vi "ATM.vi"() -> ()   [LabVIEW 2021]
doc: "This is the Main VI that performs the AMT operations."
uses:
  Controls/Queue_Operation_Select.ctl
  Controls/State_Data.ctl
  Controls/Control_Reference.ctl
  Controls/File_Operation_Select.ctl
  Controls/Timer_Operation_Select.ctl
  Controls/ATM_Data.ctl
  Controls/Right_Menu_Display.ctl
  Controls/Left_Menu_Dispaly.ctl
  Controls/Notifier_Operation_Select.ctl
  Controls/ATM_Message.ctl
panel:
  in  "User_Input":string caption="User Input"
  out "Error_Out":errorcluster
  in  "Error_In":errorcluster
  out "ATM_Message":string caption="ATM Message"
  out "Right_Menu":T1 caption="Right Menu"
  out "Left_Menu":T2 caption="Left Menu"
  in  "Right_Buttons":T3 caption="Right Buttons"
  in  "Left_Buttons":T4 caption="Left Buttons"
  in  "Enter":bool
  in  "Card_Simulator":bool caption="Card Simulator"
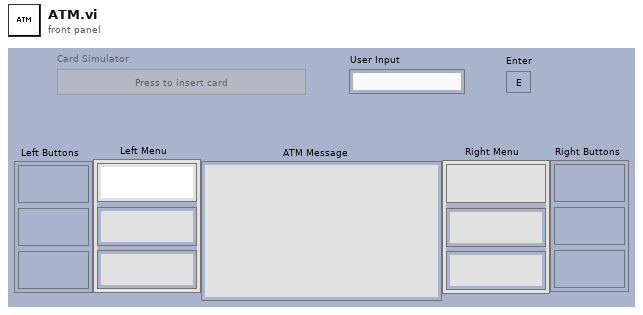
[diagram p1: front panel]
types:
  T1 = typedef "Right_Menu_Display.ctl" = cluster{"Withdraw_D":string, "Deposit_D":string, "Fast_cash_$50_D":string}
  T2 = typedef "Left_Menu_Dispaly.ctl" = cluster{"Balance_Inquiry_D":string, "None_D":string, "Return_Card_&_Terminate":string}
  T3 = cluster{"Deposit":bool, "Withdraw":bool, "Fast_Cash_$50":bool}
  T4 = cluster{"None":bool, "Balance_Inquiry":bool, "Return_Card_&_Terminate":bool}
  T5 = typedef "Notifier_Operation_Select.ctl" = enum16{"Obtain_Notification", "Send_Notification", "Get_Notification_Status", "Release_Notification"}
  T6 = typedef "Queue_Operation_Select.ctl" = enum16{"Obtain_Queue", "Enqueue", "Enqueue_N", "Enqueue_at_First", "Dequeue", "Flush_Queue", "Release_Queue"}
  T7 = typedef "Timer_Operation_Select.ctl" = enum16{"Start_Timer", "Time_Out?", "Stop_Timer"}
  T8 = typedef "State_Data.ctl" = cluster{"State":string, "Data":string}
  T9 = typedef "ATM_Data.ctl" = cluster{"Account_Details":string[][], "Selected_Account_Details":string[], "ATM_Message":string, "Left_Menu":T2, "Right_Menu":T1, "Contol_Buttons":refnum<vi>[], "Enter_&_User_Input":refnum<vi>[], "Card_Simulator":refnum<vi>[], "Disable_Control_Reference":refnum<vi>[], "Enable_Control_Reference":refnum<vi>[], "Control_Reference":T10, "Current_Process":string, "Event_Data":string, "Current_Banking_Process":string, "Selected_Banking":string, "Index_of_Selected_Account":i32, "Terminated?":bool, "Account_File_Path":path, "ATM_Message 2":T11}
  T10 = typedef "Control_Reference.ctl" = cluster{"User_Input":refnum<vi>, "Fast_Cash_$50":refnum<vi>, "Withdraw":refnum<vi>, "Deposit":refnum<vi>, "Return_Card_&_Terminate":refnum<vi>, "Balance_Inquiry":refnum<vi>, "None":refnum<vi>, "Enter":refnum<vi>, "Card_Simulator":refnum<vi>}
  T11 = typedef "ATM_Message.ctl" = cluster{"LM_Balance_Inquiry":string, "LM_None":string, "LM_Return_Card_&_Terminate":string, "RM_Withdraw":string, "RM_Deposit":string, "RM_Fast_Cash_$50":string, "ATMM_Re_Enter_AN":string, "ATMM_Home":string, "ATMM_Deposit":string, "ATMM_Withdraw":string, "ATMM_Termination":string, "ATMM_Insufficient":string, "ATMM_Balance_Inquiry":string, "ATMM_Deposit":string, "ATMM_Withdraw":string, "ATMM_Dollar":string, "ATMM_Welcome":string, "ATMM_User_Welcome":string, "ATMM_Deposit_Insufficient":string}
  T12 = typedef "File_Operation_Select.ctl" = enum16{"Get_Details", "Update_Details"}
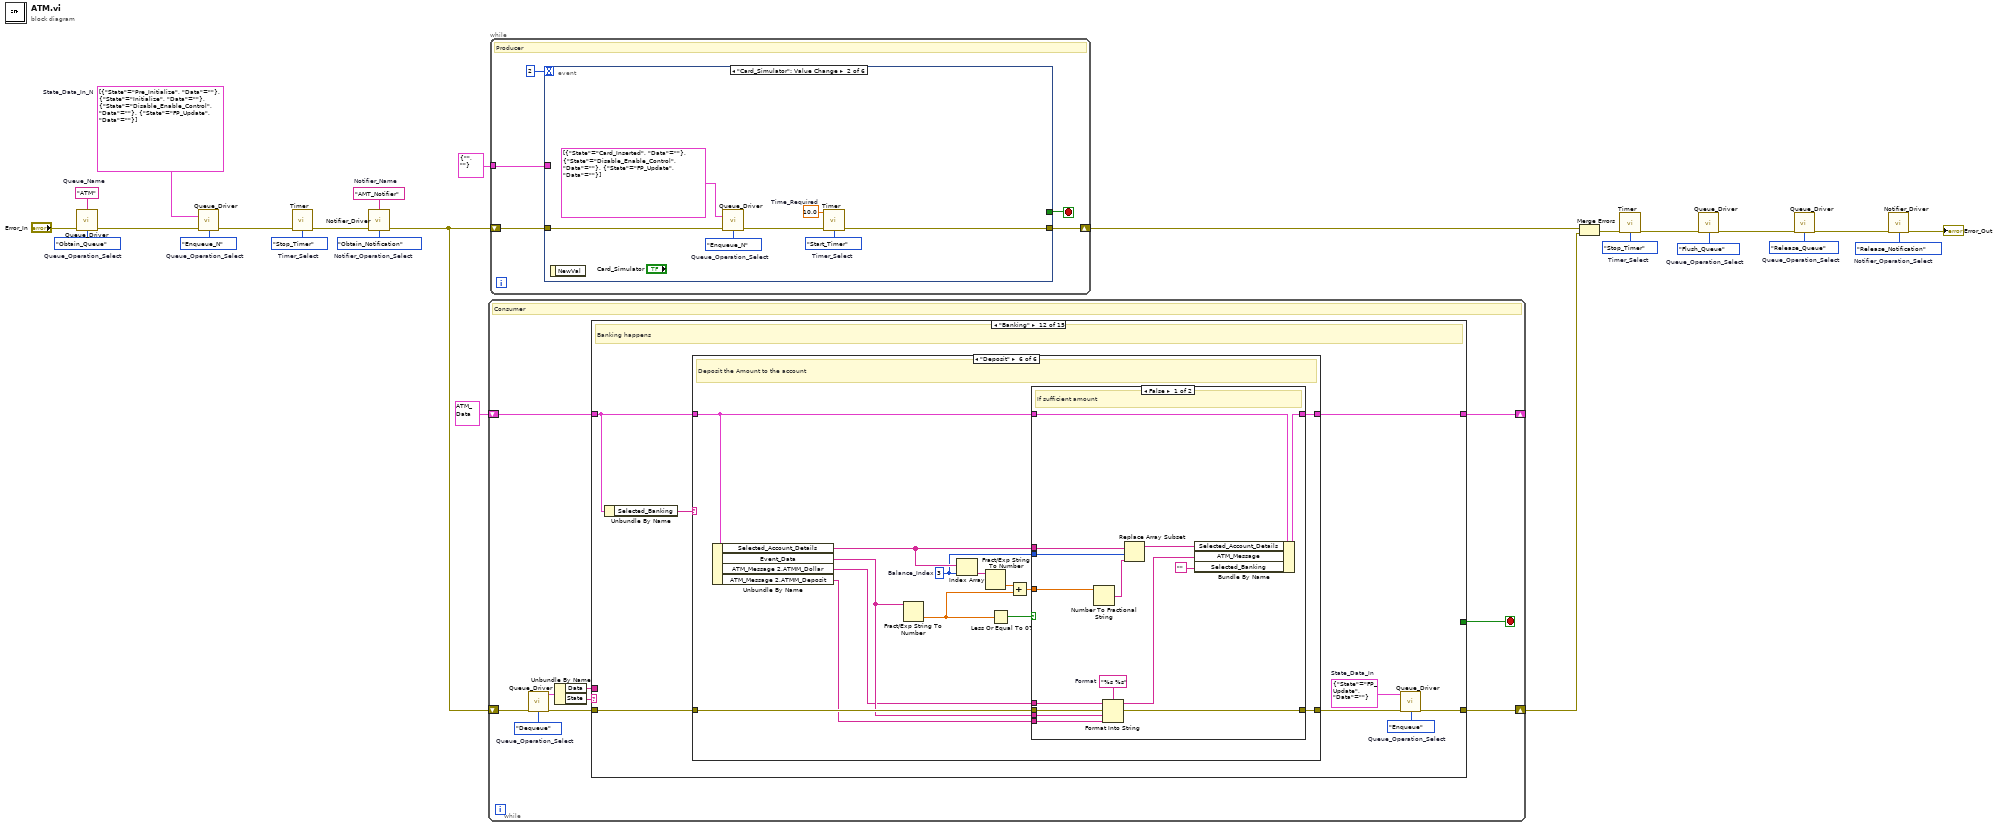
[diagram p0: block diagram]
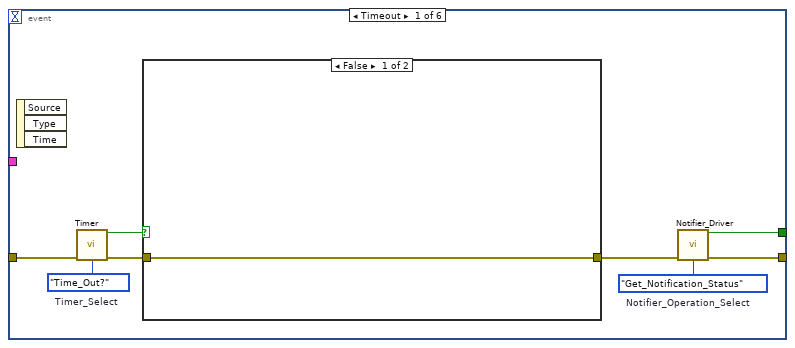
[diagram p2: hidden frame]
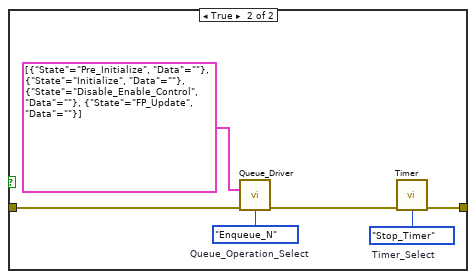
[diagram p3: hidden frame]
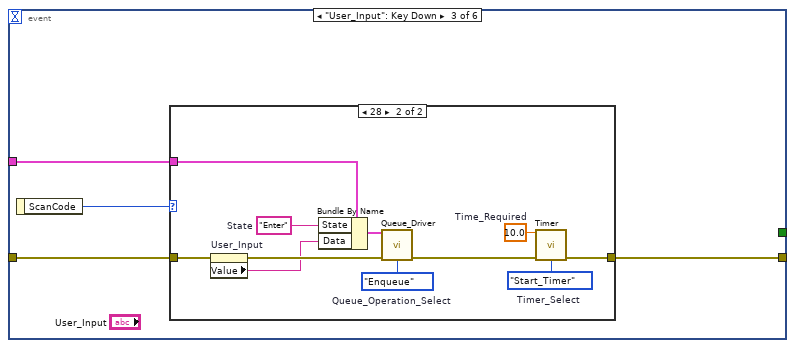
[diagram p4: hidden frame]
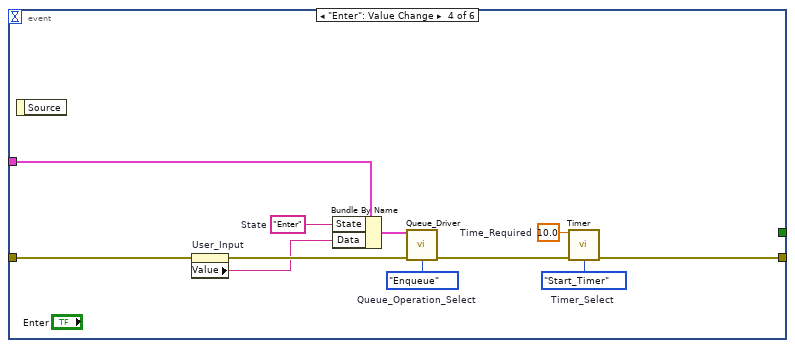
[diagram p6: hidden frame]
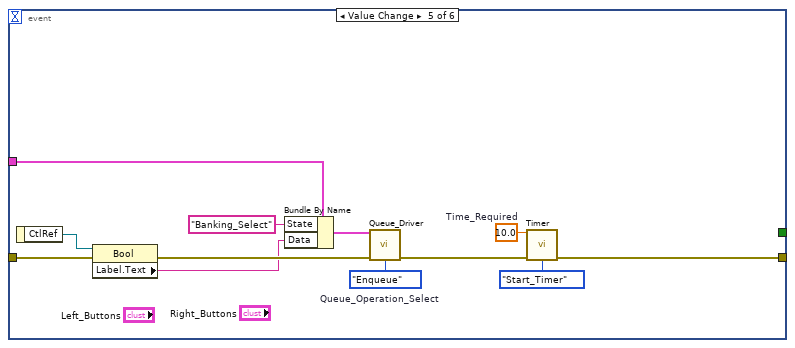
[diagram p7: hidden frame]
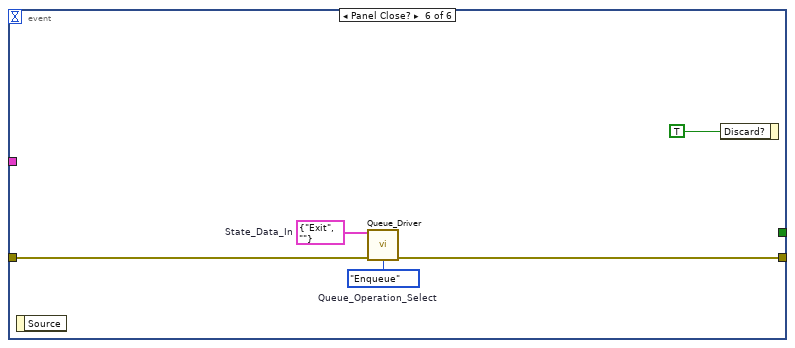
[diagram p8: hidden frame]
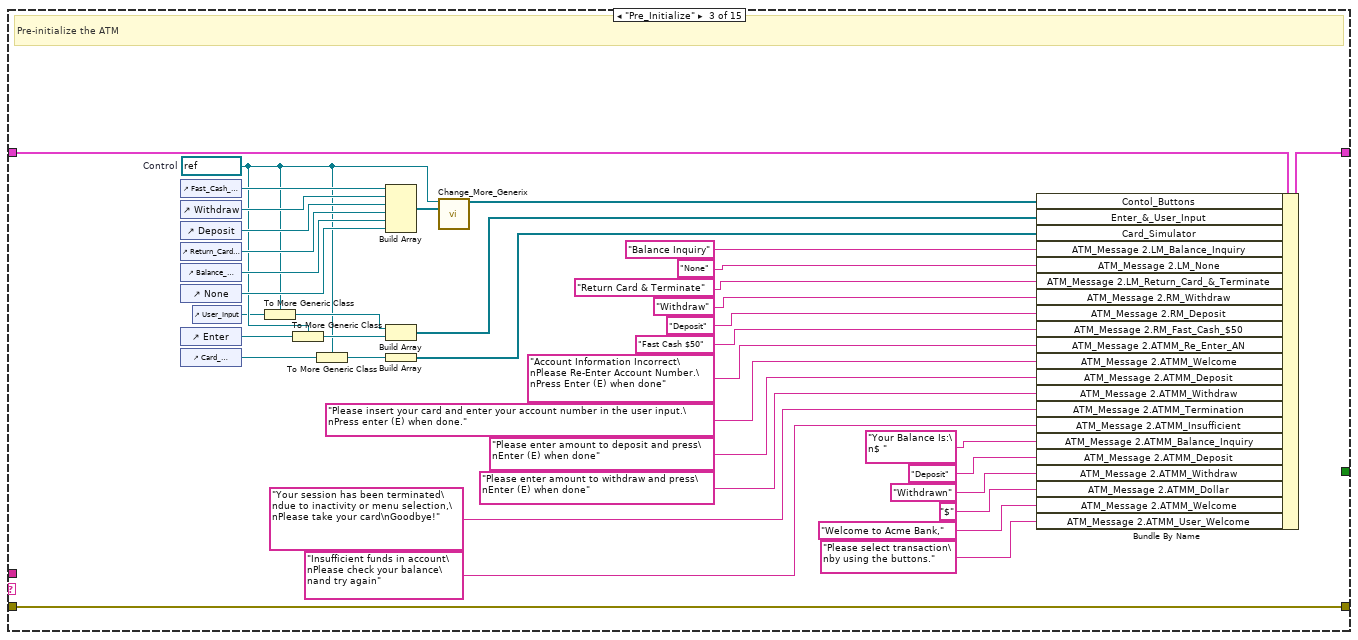
[diagram p11: hidden frame]
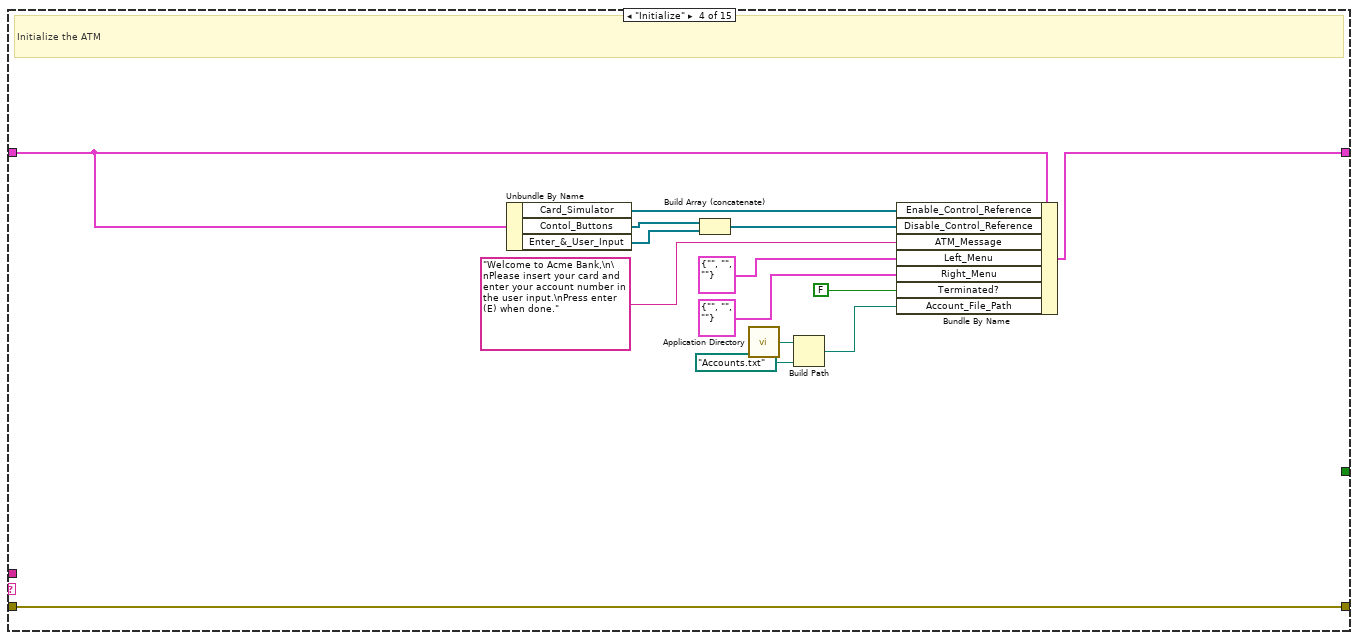
[diagram p12: hidden frame]
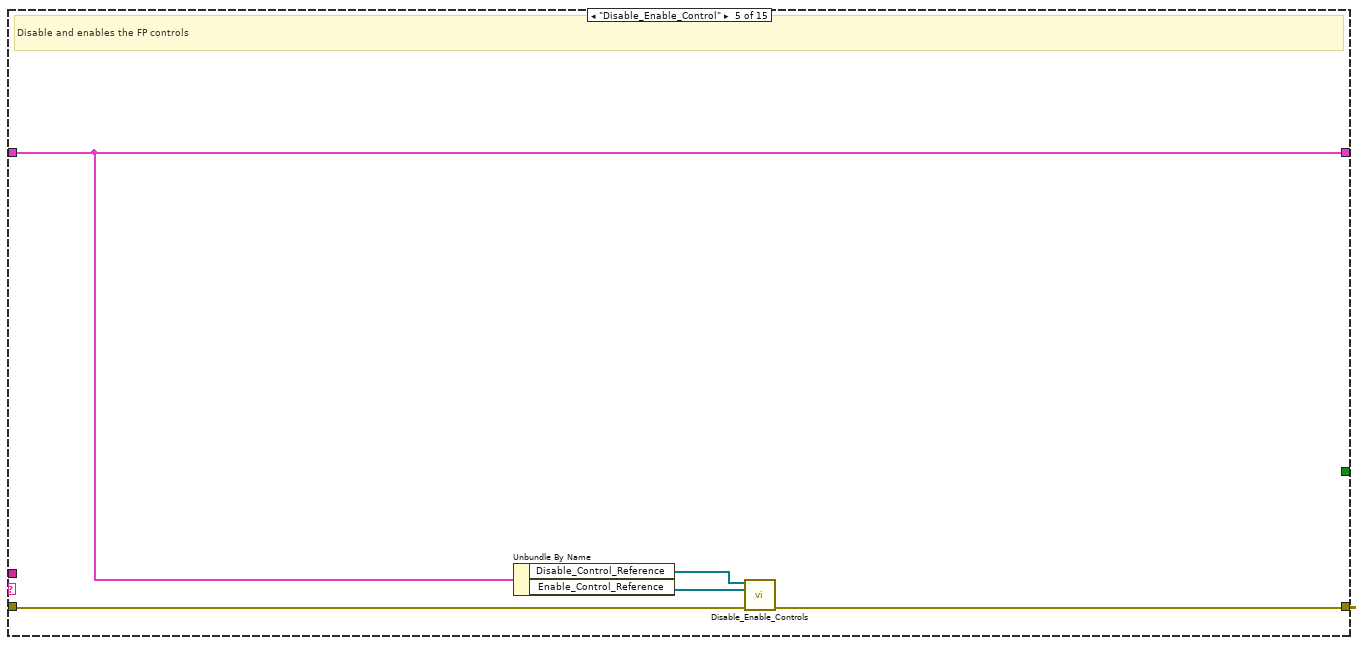
[diagram p13: hidden frame]
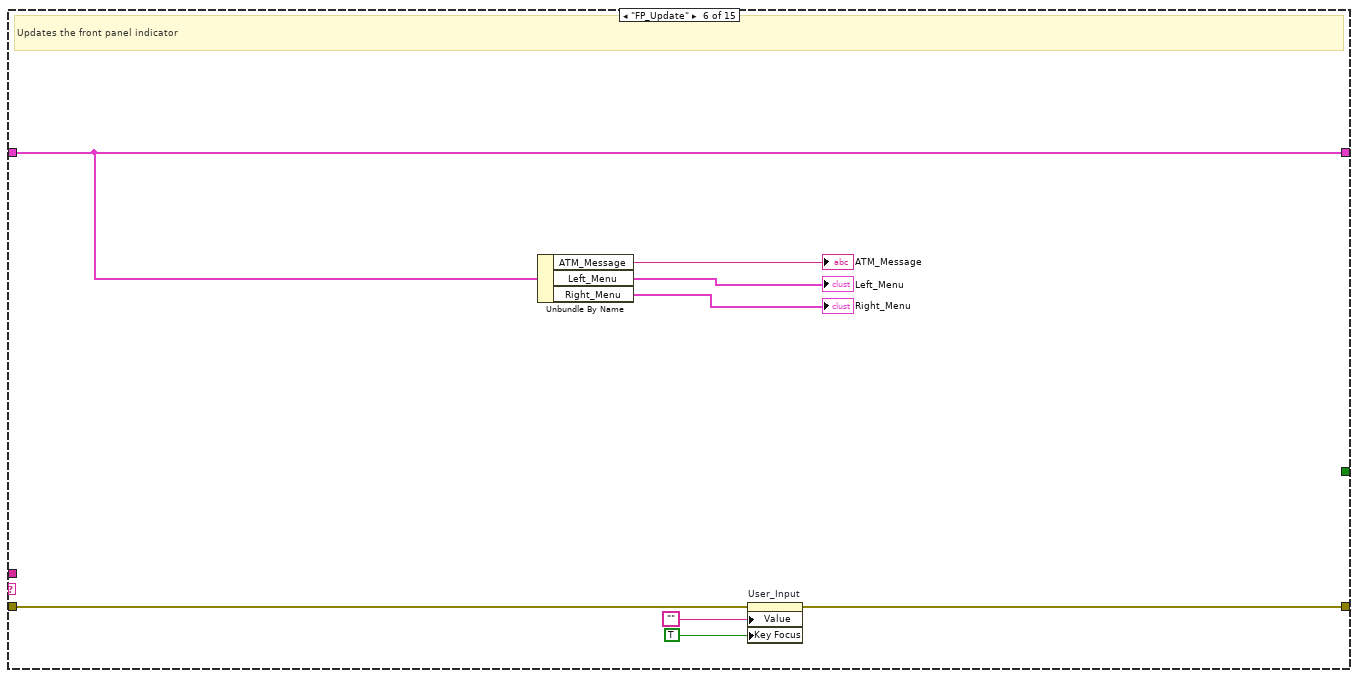
[diagram p14: hidden frame]
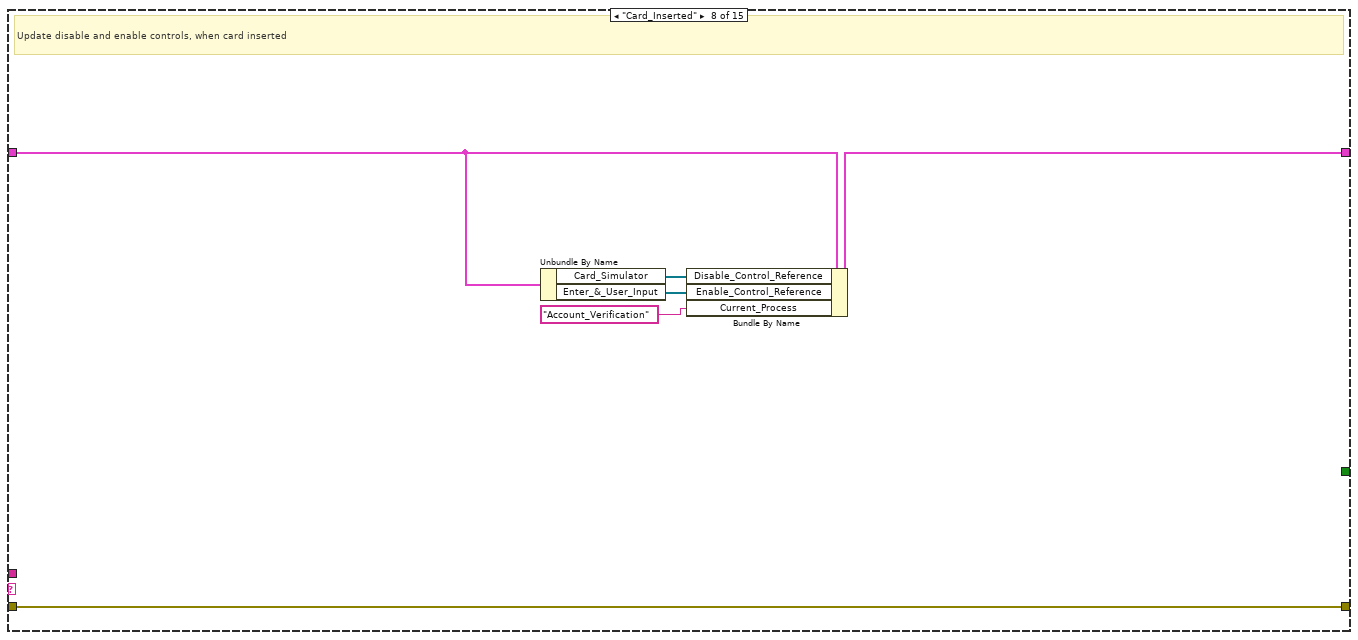
[diagram p16: hidden frame]
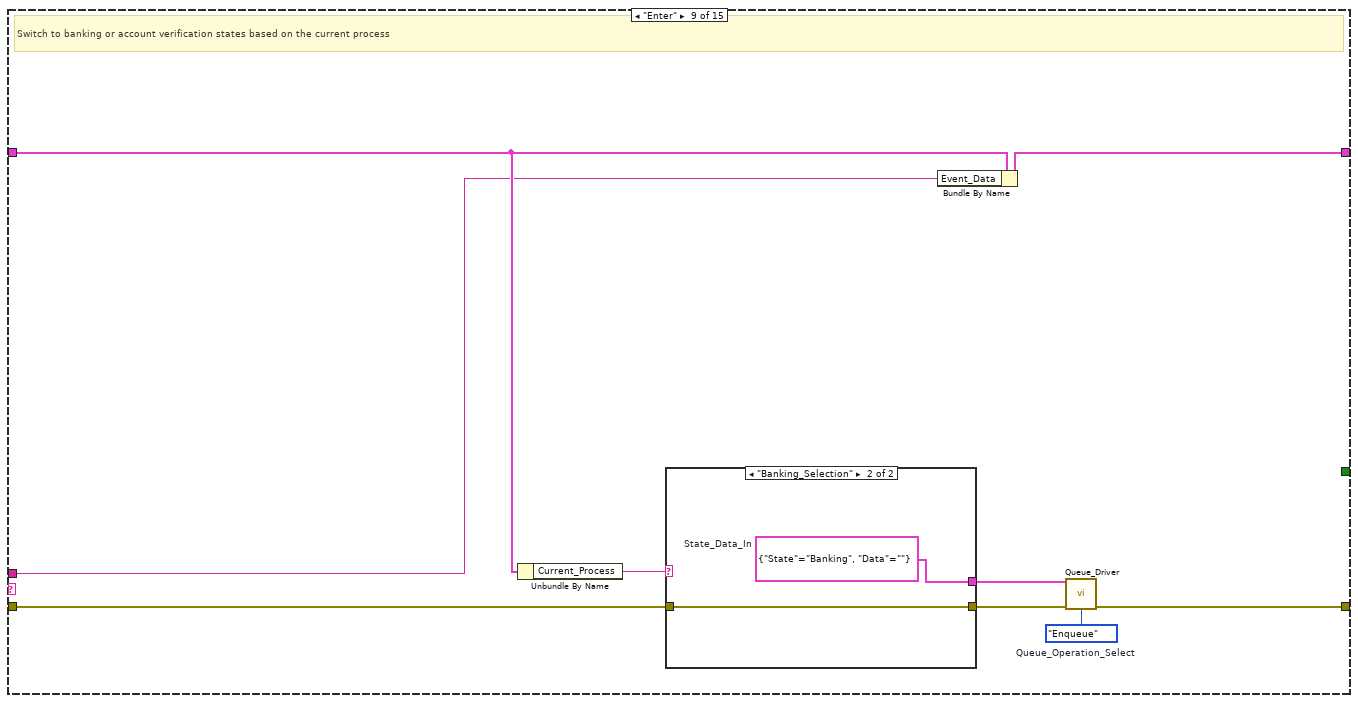
[diagram p17: hidden frame]
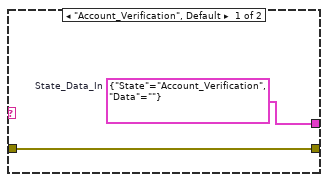
[diagram p18: hidden frame]
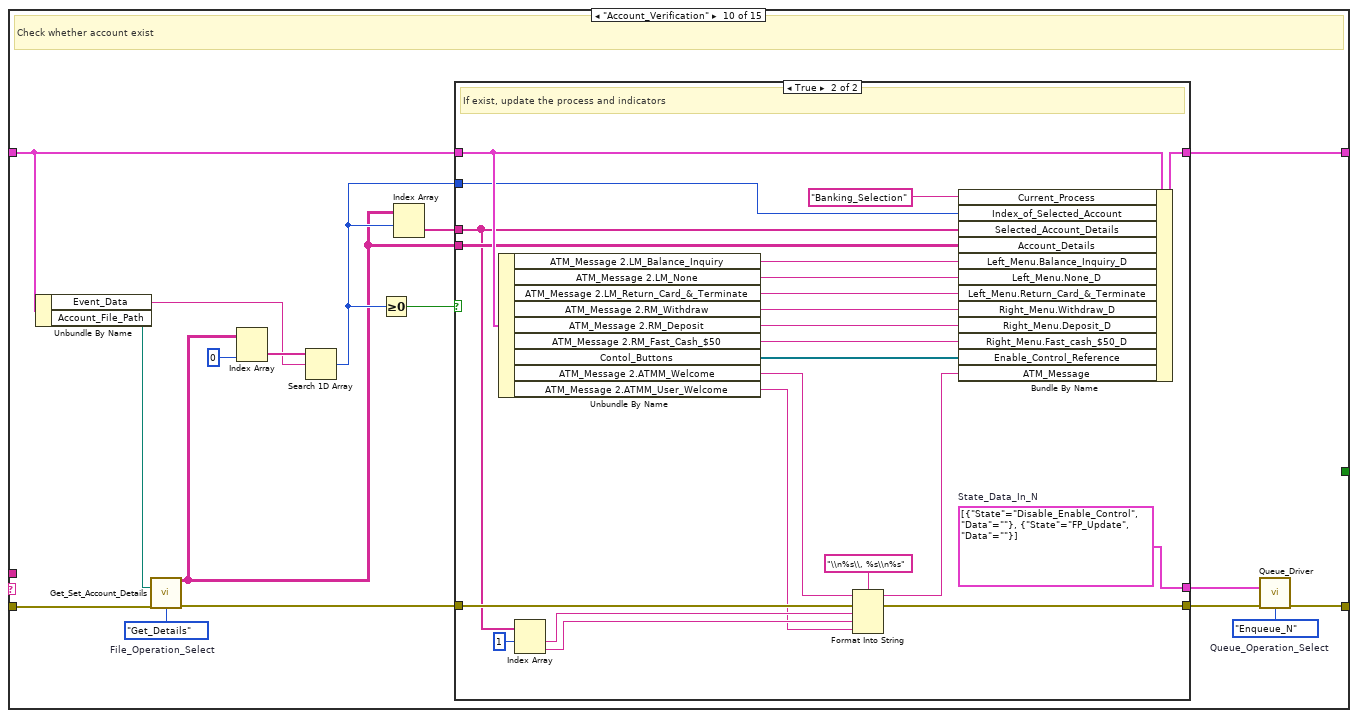
[diagram p19: hidden frame]
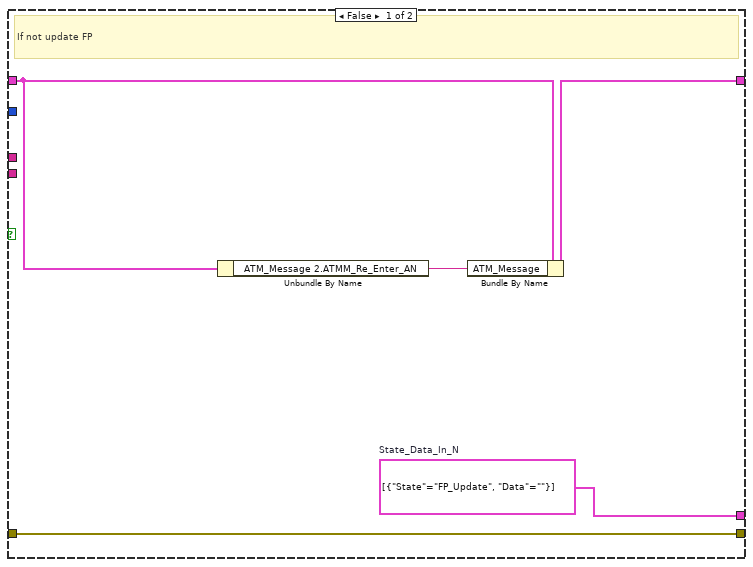
[diagram p20: hidden frame]
diagram:
  w4 = Notifier_Operation_Select."Release_Notification"  # Notifier_Operation_Select
  w5 = Queue_Operation_Select."Release_Queue"  # Queue_Operation_Select
  w7 = Queue_Operation_Select."Flush_Queue"  # Queue_Operation_Select
  w8 = Timer_Operation_Select."Stop_Timer"  # Timer_Select
  w11 = "AMT_Notifier"  # Notifier_Name
  w12 = Notifier_Operation_Select."Obtain_Notification"  # Notifier_Operation_Select
  w15 = Timer_Operation_Select."Stop_Timer"  # Timer_Select
  w18 = T8[] [{"State"="Pre_Initialize", "Data"=""}, {"State"="Initialize", "Data"=""}, {"State"="Disable_Enable_Control", "Data"=""}, {"State"="FP_Update", "Data"=""}]  # State_Data_In_N
  w19 = Queue_Operation_Select."Enqueue_N"  # Queue_Operation_Select
  w22 = "ATM"  # Queue_Name
  w23 = Queue_Operation_Select."Obtain_Queue"  # Queue_Operation_Select
  n1 = call "Queue_Driver.vi"("Queue_Name"=w22, "Error_In"="Error_In", "Queue_Operation_Select"=w23) -> ("Error_Out"=w24:errorcluster)  [unwired: 11 in, 1 out]
  n2 = call "Queue_Driver.vi"("State_Data_In_N"=w18, "Error_In"=w24, "Queue_Operation_Select"=w19) -> ("Error_Out"=w20:errorcluster)  [unwired: 11 in, 1 out]
  n3 = call "Timer.vi"("Error_In"=w20, "Timer_Select"=w15) -> ("Error_Out"=w16:errorcluster)  [unwired: 12 in, 1 out]
  n4 = call "Notifier_Driver.vi"("Notifier_Name"=w11, "Error_In"=w16, "Notifier_Operation_Select"=w12) -> ("Error_Out"=w13:errorcluster)  [unwired: 11 in, 1 out]
  n5 = while {
    shift-right: [w28] -> _
    shift-left: T9 {"Account_Details"=[], "Selected_Account_Details"=[], "ATM_Message"="", "Left_Menu"={"Balance_Inquiry_D"="", "None_D"="", "Return_Card_&_Terminate"=""}, "Right_Menu"={"Withdraw_D"="", "Deposit_D"="", "Fast_cash_$50_D"=""}, "Contol_Buttons"=[], "Enter_&_User_Input"=[], "Card_Simulator"=[], "Disable_Control_Reference"=[], "Enable_Control_Reference"=[], "Control_Reference"={"User_Input"=refnum, "Fast_Cash_$50"=refnum, "Withdraw"=refnum, "Deposit"=refnum, "Return_Card_&_Terminate"=refnum, "Balance_Inquiry"=refnum, "None"=refnum, "Enter"=refnum, "Card_Simulator"=refnum}, "Current_Process"="", "Event_Data"="", "Current_Banking_Process"="", "Selected_Banking"="", "Index_of_Selected_Account"=0, "Terminated?"=FALSE, "Account_File_Path"=path "", "ATM_Message 2"={"LM_Balance_Inquiry"="", "LM_None"="", "LM_Return_Card_&_Terminate"="", "RM_Withdraw"="", "RM_Deposit"="", "RM_Fast_Cash_$50"="", "ATMM_Re_Enter_AN"="", "ATMM_Home"="", "ATMM_Deposit"="", "ATMM_Withdraw"="", "ATMM_Termination"="", "ATMM_Insufficient"="", "ATMM_Balance_Inquiry"="", "ATMM_Deposit"="", "ATMM_Withdraw"="", "ATMM_Dollar"="", "ATMM_Welcome"="", "ATMM_User_Welcome"="", "ATMM_Deposit_Insufficient"=""}} -> [w29]
    shift-right: [w34] -> w14
    shift-left: w13 -> [w35]
    stop <- w26 stop-if-true
    w32 = Queue_Operation_Select."Dequeue"  # Queue_Operation_Select
    # "Consumer"
    n6 = call "Queue_Driver.vi"("Error_In"=w35, "Queue_Operation_Select"=w32) -> ("State_Data_Out"=w30:T8, "Error_Out"=w33:errorcluster)  [unwired: 12 in]
    n7 = Unbundle By Name(w30) -> ("Data"=w27:string, "State"=w31:string)
    n8 = case shown="\"Banking\"" w31 {
      tunnel: w33 -> [w37 w39 w77 w91 w96 w102 w106 w107 w120 w142 w185 w223 w326 w333 w350]
      tunnel: [w37 w39 w77 w91 w95 w101 w106 w107 w115 w132 w178 w218 w326 w332 w352] -> w34
      tunnel: w29 -> [w36 w38 w76 w90 w92 w104 w105 w111 w118 w140 w171 w221 w325 w344 w353]
      tunnel: [w36 w38 w75 w89 w92 w104 w105 w112 w117 w136 w184 w224 w325 w344 w353] -> w28
      tunnel: w27 -> [_ _ _ _ _ _ _ _ w116 _ w182 _ _ _ _]
      tunnel: [_ _ _ _ _ _ _ _ _ _ _ _ _ _ w345] -> w26
      frame Default {
        # "Default"
      }
      frame "---Initialize_and_Update_Front_Panel---" {
        # "States after this are initialization and front panel updation"
      }
      frame "Pre_Initialize" {
        w60 = refnum<vi> refnum  # Control
        # "Pre-initialize the ATM"
        n9 = control-ref of="Fast_Cash_$50"() -> (w74:refnum<vi>)
        n10 = control-ref of="Withdraw"() -> (w73:refnum<vi>)
        n11 = control-ref of="Deposit"() -> (w72:refnum<vi>)
        n12 = control-ref of="Return_Card_&_Terminate"() -> (w71:refnum<vi>)
        n13 = control-ref of="Balance_Inquiry"() -> (w70:refnum<vi>)
        n14 = control-ref of="None"() -> (w65:refnum<vi>)
        n15 = control-ref of="Enter"() -> (w67:refnum<vi>)
        n16 = control-ref of="Card_Simulator"() -> (w59:refnum<vi>)
        n17 = control-ref of="User_Input"() -> (w58:refnum<vi>)
        n18 = To More Generic Class(target class=w60, reference=w58) -> (generic class reference=w66:refnum<vi>)
        n19 = To More Generic Class(target class=w60, reference=w67) -> (generic class reference=w63:refnum<vi>)
        n20 = To More Generic Class(target class=w60, reference=w59) -> (generic class reference=w61:refnum<vi>)
        n21 = Build Array(w74, w73, w72, w71, w70, w65) -> (w69:refnum<vi>[])
        n22 = Build Array(w66, w63) -> (w64:refnum<vi>[])
        n23 = Build Array(w61) -> (w62:refnum<vi>[])
        n24 = call "Change_More_Generix.vi"("Control_In"=w60, "Reference_In"=w69) -> ("Reference_Out"=w68:refnum<vi>[])  [unwired: 13 in]
        n25 = Bundle By Name(cluster=w76, "Contol_Buttons"=w68, "Enter_&_User_Input"=w64, "Card_Simulator"=w62, "ATM_Message 2.LM_Balance_Inquiry"="Balance Inquiry" ("Left_Menu.Balance_Inquiry_D"), "ATM_Message 2.LM_None"="None" ("Left_Menu.None_D"), "ATM_Message 2.LM_Return_Card_&_Terminate"="Return Card & Terminate" ("Left_Menu.Return_Card_&_Terminate"), "ATM_Message 2.RM_Withdraw"="Withdraw" ("Right_Menu.Withdraw_D"), "ATM_Message 2.RM_Deposit"="Deposit" ("Right_Menu.Deposit_D"), "ATM_Message 2.RM_Fast_Cash_$50"="Fast Cash $50" ("Right_Menu.Fast_cash_$50_D"), "ATM_Message 2.ATMM_Re_Enter_AN"="Account Information Incorrect\nPlease Re-Enter Account Number.\nPress Enter (E) when done", "ATM_Message 2.ATMM_Welcome"="Please insert your card and enter your account number in the user input.\nPress enter (E) when done." ("ATM_Message"), "ATM_Message 2.ATMM_Deposit"="Please enter amount to deposit and press\nEnter (E) when done", "ATM_Message 2.ATMM_Withdraw"="Please enter amount to withdraw and press\nEnter (E) when done", "ATM_Message 2.ATMM_Termination"="Your session has been terminated\ndue to inactivity or menu selection,\nPlease take your card\nGoodbye!" ("ATM_Message"), "ATM_Message 2.ATMM_Insufficient"="Insufficient funds in account\nPlease check your balance\nand try again" ("ATM_Message"), "ATM_Message 2.ATMM_Balance_Inquiry"="Your Balance Is:\n$ " ("Message"), "ATM_Message 2.ATMM_Deposit"="Deposit", "ATM_Message 2.ATMM_Withdraw"="Withdrawn", "ATM_Message 2.ATMM_Dollar"="$", "ATM_Message 2.ATMM_Welcome"="Welcome to Acme Bank,", "ATM_Message 2.ATMM_User_Welcome"="Please select transaction\nby using the buttons.") -> (w75:T9)
      }
      frame "Initialize" {
        # "Initialize the ATM"
        n26 = Unbundle By Name(w90) -> ("Card_Simulator"=w84:refnum<vi>[], "Contol_Buttons"=w88:refnum<vi>[], "Enter_&_User_Input"=w87:refnum<vi>[])
        n27 = Build Array (concatenate)(w88, w87) -> (w86:refnum<vi>[])
        n28 = call <vilib>:"Application Directory.vi"() -> ("Application Directory"=w79:path)
        n29 = Build Path(base path=w79, name or relative path=path "Accounts.txt") -> (appended path=w78:path)
        n30 = Bundle By Name(cluster=w90, "Enable_Control_Reference"=w84, "Disable_Control_Reference"=w86, "ATM_Message"="Welcome to Acme Bank,\n\nPlease insert your card and enter your account number in the user input.\nPress enter (E) when done.", "Left_Menu"=T2 {"Balance_Inquiry_D"="", "None_D"="", "Return_Card_&_Terminate"=""}, "Right_Menu"=T1 {"Withdraw_D"="", "Deposit_D"="", "Fast_cash_$50_D"=""}, "Terminated?"=FALSE, "Account_File_Path"=w78) -> (w89:T9)
      }
      frame "Disable_Enable_Control" {
        # "Disable and enables the FP controls"
        n31 = Unbundle By Name(w92) -> ("Disable_Control_Reference"=w94:refnum<vi>[], "Enable_Control_Reference"=w93:refnum<vi>[])
        n32 = call "Disable_Enable_Controls.vi"("Disable_Control"=w94, "Enable_Control"=w93, "Error_In"=w96) -> ("Error_Out"=w95:errorcluster)  [unwired: 12 in]
      }
      frame "FP_Update" {
        # "Updates the front panel indicator"
        n33 = Unbundle By Name(w104) -> ("ATM_Message"=→"ATM_Message":string, "Left_Menu"=→"Left_Menu":T2, "Right_Menu"=→"Right_Menu":T1)
        n34 = property on="User_Input" class="Str"(error in=w102, "Value"="" ("User_Input"), "Key Focus"=TRUE) -> (error out=w101:errorcluster)  [unwired: 1 in, 1 out]
      }
      frame "-------------Banking_States-------------" {
        # "States after this are Banking stats"
      }
      frame "Card_Inserted" {
        # "Update disable and enable controls, when card inserted"
        n35 = Unbundle By Name(w111) -> ("Card_Simulator"=w109:refnum<vi>[], "Enter_&_User_Input"=w110:refnum<vi>[])
        n36 = Bundle By Name(cluster=w111, "Disable_Control_Reference"=w109, "Enable_Control_Reference"=w110, "Current_Process"="Account_Verification") -> (w112:T9)
      }
      frame "Enter" {
        w114 = Queue_Operation_Select."Enqueue"  # Queue_Operation_Select
        # "Switch to banking or account verification states based on the current process"
        n37 = Unbundle By Name(w118) -> ("Current_Process"=w121:string)
        n38 = case shown="\"Banking_Selection\"" w121 {
          tunnel: w120 -> [w123 w125]
          tunnel: [w123 w125] -> w119
          tunnel: [w122 w124] -> w113
          frame "Account_Verification", Default {
            w122 = T8 {"State"="Account_Verification", "Data"=""}  # State_Data_In
          }
          frame "Banking_Selection" {
            w124 = T8 {"State"="Banking", "Data"=""}  # State_Data_In
          }
        }
        n39 = Bundle By Name(cluster=w118, "Event_Data"=w116) -> (w117:T9)
        n40 = call "Queue_Driver.vi"("State_Data_In"=w113, "Error_In"=w119, "Queue_Operation_Select"=w114) -> ("Error_Out"=w115:errorcluster)  [unwired: 11 in, 1 out]
      }
      frame "Account_Verification" {
        w131 = Queue_Operation_Select."Enqueue_N"  # Queue_Operation_Select
        w141 = File_Operation_Select."Get_Details"  # File_Operation_Select
        # "Check whether account exist"
        n41 = Unbundle By Name(w140) -> ("Event_Data"=w137:string, "Account_File_Path"=w129:path)
        n42 = call "Get_Set_Account_Details.vi"("File_Path"=w129, "error in (no error)"=w142, "File_Operation_Select"=w141) -> ("Account_Details"=w127:string[][], "error out"=w135:errorcluster)  [unwired: 11 in]
        n43 = Index Array(array=w127, index (col)=0 ("disabled index (col)")) -> (element=w138:string[])  [unwired: 1 in]
        n44 = Search 1D Array(1D array=w138, element=w137) -> (index of element=w128:i32)  [unwired: 1 in]
        n45 = Greater Or Equal To 0?(x=w128) -> (x >= 0?=w134:bool)
        n46 = Index Array(array=w127, index (row)=w128) -> (element=w126:string[])  [unwired: 1 in]
        n47 = case shown="True" w134 {
          tunnel: w140 -> [w144 w168]
          tunnel: [w146 w170] -> w136
          tunnel: w135 -> [w147 w169]
          tunnel: [w147 w166] -> w133
          tunnel: [w145 w160] -> w130
          tunnel: w128 -> [_ w153]
          tunnel: w127 -> [_ w152]
          tunnel: w126 -> [_ w151]
          frame False {
            w145 = T8[] [{"State"="FP_Update", "Data"=""}]  # State_Data_In_N
            # "If not update FP"
            n48 = Unbundle By Name(w144) -> ("ATM_Message 2.ATMM_Re_Enter_AN"=w143:string)
            n49 = Bundle By Name(cluster=w144, "ATM_Message"=w143) -> (w146:T9)
          }
          frame True {
            w160 = T8[] [{"State"="Disable_Enable_Control", "Data"=""}, {"State"="FP_Update", "Data"=""}]  # State_Data_In_N
            # "If exist, update the process and indicators"
            n50 = Unbundle By Name(w168) -> ("ATM_Message 2.LM_Balance_Inquiry"=w156:string, "ATM_Message 2.LM_None"=w155:string, "ATM_Message 2.LM_Return_Card_&_Terminate"=w154:string, "ATM_Message 2.RM_Withdraw"=w157:string, "ATM_Message 2.RM_Deposit"=w158:string, "ATM_Message 2.RM_Fast_Cash_$50"=w159:string, "Contol_Buttons"=w167:refnum<vi>[], "ATM_Message 2.ATMM_Welcome"=w150:string, "ATM_Message 2.ATMM_User_Welcome"=w149:string)
            n51 = Index Array(array=w151, index #1=1 ("index")) -> (element #1=w163:string, element #2=w161:string)  [unwired: 1 in]
            n52 = Format Into String(format string="\\n%s\\, %s\\n%s", initial string=w150, error in=w169, w163, w161, w149) -> (resulting string=w165:string, error out=w166:errorcluster)
            n53 = Bundle By Name(cluster=w168, "Current_Process"="Banking_Selection", "Index_of_Selected_Account"=w153, "Selected_Account_Details"=w151, "Account_Details"=w152, "Left_Menu.Balance_Inquiry_D"=w156, "Left_Menu.None_D"=w155, "Left_Menu.Return_Card_&_Terminate"=w154, "Right_Menu.Withdraw_D"=w157, "Right_Menu.Deposit_D"=w158, "Right_Menu.Fast_cash_$50_D"=w159, "Enable_Control_Reference"=w167, "ATM_Message"=w165) -> (w170:T9)
          }
        }
        n54 = call "Queue_Driver.vi"("State_Data_In_N"=w130, "Error_In"=w133, "Queue_Operation_Select"=w131) -> ("Error_Out"=w132:errorcluster)  [unwired: 11 in, 1 out]
      }
      frame "Banking_Select" {
        w174 = ""  # Default
        w177 = Queue_Operation_Select."Enqueue_N"  # Queue_Operation_Select
        # "Updates the Banking Selected"
        n55 = Unbundle By Name(w171) -> ("Terminated?"=w175:bool)
        n56 = Select(t=w174, s=w175, f=w182) -> (s? t:f=w176:string)
        n57 = case shown="Default" w176 {
          selector: w176 -> [w188 w192 w196 w200 w205 w210 _]
          tunnel: w185 -> [w189 w193 w197 w201 w206 w211 w216]
          tunnel: [w189 w193 w197 w201 w206 w211 w216] -> w179
          tunnel: [_ _ _ _ w202 w207 _] -> w183
          tunnel: [_ _ _ _ _ _ "50" ("Event_Data")] -> w181
          tunnel: [w188 w192 w196 w200 w205 w210 "Withdraw"] -> w180
          tunnel: [w187 T8[] [{"State"="Banking", "Data"=""}] ("State_Data_In") T8[] [{"State"="Banking", "Data"=""}] ("State_Data_In") w198 w204 w209 T8[] [{"State"="Banking", "Data"=""}] ("State_Data_In")] -> w173
          tunnel: [w186 w191 w195 w199 w203 w208 w213] -> w172
          tunnel: w171 -> [w186 w191 w195 w199 w203 w208 w213]
          frame Default {
            w187 = T8[] [{"State"="Pre_Initialize", "Data"=""}, {"State"="Initialize", "Data"=""}, {"State"="Disable_Enable_Control", "Data"=""}, {"State"="FP_Update", "Data"=""}]  # State_Data_In_N
            # "Re initialize, if terminated and button pressed"
          }
          frame "Return_Card_&_Terminate" {
            # "Terminate the session"
          }
          frame "Balance_Inquiry" {
            # "Switch to Banking and get the balance"
          }
          frame "None" {
            w198 = T8[] []  # State_Data_In
            # "#Future updates"
          }
          frame "Deposit" {
            w204 = T8[] [{"State"="FP_Update", "Data"=""}]  # State_Data_In
            # "Update FP and with for Amount enter"
            n58 = Unbundle By Name(w203) -> ("ATM_Message 2.ATMM_Deposit"=w202:string)
          }
          frame "Withdraw" {
            w209 = T8[] [{"State"="FP_Update", "Data"=""}]  # State_Data_In
            # "Update FP and wait for withdraw amount"
            n59 = Unbundle By Name(w208) -> ("ATM_Message 2.ATMM_Withdraw"=w207:string)
          }
          frame "Fast_Cash_$50" {
            # "Switch to banking and debit 50"
          }
        }
        n60 = Bundle By Name(cluster=w172, "ATM_Message"=w183, "Event_Data"=w181, "Selected_Banking"=w180) -> (w184:T9)
        n61 = call "Queue_Driver.vi"("State_Data_In_N"=w173, "Error_In"=w179, "Queue_Operation_Select"=w177) -> ("Error_Out"=w178:errorcluster)  [unwired: 11 in, 1 out]
      }
      frame "Banking" {
        w219 = T8 {"State"="FP_Update", "Data"=""}  # State_Data_In
        w220 = Queue_Operation_Select."Enqueue"  # Queue_Operation_Select
        # "Banking happens"
        n62 = Unbundle By Name(w221) -> ("Selected_Banking"=w217:string)
        n63 = case shown="\"Deposit\"" w217 {
          tunnel: w221 -> [w226 w241 w250 w253 w261 w303]
          tunnel: [w239 w242 w246 w253 w262 w304] -> w224
          tunnel: w223 -> [w237 w243 w251 w252 w263 w305]
          tunnel: [w232 w243 w251 w252 w264 w297] -> w222
          frame "Return_Card_&_Terminate" {
            w230 = 3.0  # Time_Required
            w231 = Timer_Operation_Select."Start_Timer"  # Timer_Select
            w238 = File_Operation_Select."Update_Details"  # File_Operation_Select
            # "Terminate the session"
            n64 = Unbundle By Name(w226) -> ("ATM_Message 2.ATMM_Termination"=w225:string, "Account_Details"=w236:string[][], "Index_of_Selected_Account"=w235:i32, "Selected_Account_Details"=w234:string[], "Account_File_Path"=w227:path)
            n65 = Replace Array Subset(array=w236, new element=w234, index (row)=w235) -> (w233:string[][])  [unwired: 1 in]
            n66 = call "Get_Set_Account_Details.vi"("Updated_Account_Details"=w233, "File_Path"=w227, "error in (no error)"=w237, "File_Operation_Select"=w238) -> ("error out"=w229:errorcluster)  [unwired: 10 in, 1 out]
            n67 = Bundle By Name(cluster=w226, "ATM_Message"=w225, "Terminated?"=TRUE) -> (w239:T9)
            n68 = call "Timer.vi"("Time_Required"=w230, "Error_In"=w229, "Timer_Select"=w231) -> ("Error_Out"=w232:errorcluster)  [unwired: 11 in, 1 out]
          }
          frame Default {
            n69 = Unbundle By Name(w241) -> ("ATM_Message 2.ATMM_Welcome"=w240:string)
            n70 = Bundle By Name(cluster=w241, "ATM_Message"=w240) -> (w242:T9)
          }
          frame "Balance_Inquiry" {
            w248 = 3  # Balance_Index
            # "Get the balance from the account"
            n71 = Unbundle By Name(w250) -> ("ATM_Message 2.ATMM_Balance_Inquiry"=w244:string, "Selected_Account_Details"=w249:string[])
            n72 = Index Array(array=w249, index=w248) -> (element=w247:string)
            n73 = Concatenate Strings(w244, w247) -> (w245:string)
            n74 = Bundle By Name(cluster=w250, "ATM_Message"=w245) -> (w246:T9)
          }
          frame "None" {
            # "#FutureUpdate"
          }
          frame "Withdraw" {
            w270 = 3  # Balance_Index
            # "Withdraw the Amount from account"
            n75 = Unbundle By Name(w261) -> ("Selected_Account_Details"=w268:string[], "Event_Data"=w258:string, "ATM_Message 2.ATMM_Dollar"=w260:string, "ATM_Message 2.ATMM_Withdraw"=w259:string)
            n76 = Lexical Class(1:w258) -> (0:w257:i16)
            n77 = Equal?(x=i16 3, y=w257) -> (x = y?=w254:bool)
            n78 = Index Array(array=w268, index=w270) -> (element=w269:string)
            n79 = Fract/Exp String To Number(string=w258) -> (number=w265:dbl)  [unwired: 3 in, 1 out]
            n80 = Fract/Exp String To Number(string=w269) -> (number=w266:dbl)  [unwired: 3 in, 1 out]
            n81 = Greater Or Equal?(x=w266, y=w265) -> (x >= y?=w267:bool)
            n82 = And(x=w254, y=w267) -> (x .and. y?=w255:bool)
            n83 = case shown="True" w255 {
              tunnel: w268 -> [_ w291]
              tunnel: w266 -> [_ w290]
              tunnel: w265 -> [_ w289]
              tunnel: [w274 w281] -> w264
              tunnel: w263 -> [w274 w285]
              tunnel: [w273 w283] -> w262
              tunnel: w261 -> [w272 w284]
              tunnel: w258 -> [_ w279]
              tunnel: w260 -> [_ w276]
              tunnel: w259 -> [_ w275]
              frame False {
                # "If Insufficient"
                n84 = Unbundle By Name(w272) -> ("ATM_Message 2.ATMM_Insufficient"=w271:string)
                n85 = Bundle By Name(cluster=w272, "ATM_Message"=w271) -> (w273:T9)
              }
              frame True {
                w280 = "%s %s "  # Format
                w286 = 3  # Balance_Index
                # "If Sufficient"
                n86 = Subtract(x=w290, y=w289) -> (x-y=w288:dbl)
                n87 = Number To Fractional String(number=w288) -> (F-format string=w287:string)  [unwired: 3 in]
                n88 = Replace Array Subset(array=w291, new element=w287, index=w286) -> (w282:string[])
                n89 = Format Into String(format string=w280, initial string=w276, error in=w285, w279, w275) -> (resulting string=w278:string, error out=w281:errorcluster)
                n90 = Bundle By Name(cluster=w284, "Selected_Account_Details"=w282, "ATM_Message"=w278, "Selected_Banking"="") -> (w283:T9)
              }
            }
          }
          frame "Deposit" {
            w298 = 3  # Balance_Index
            # "Deposit the Amount to the account"
            n91 = Unbundle By Name(w303) -> ("Selected_Account_Details"=w299:string[], "Event_Data"=w296:string, "ATM_Message 2.ATMM_Dollar"=w293:string, "ATM_Message 2.ATMM_Deposit"=w292:string)
            n92 = Fract/Exp String To Number(string=w296) -> (number=w295:dbl)  [unwired: 3 in, 1 out]
            n93 = Index Array(array=w299, index=w298) -> (element=w302:string)
            n94 = Fract/Exp String To Number(string=w302) -> (number=w301:dbl)  [unwired: 3 in, 1 out]
            n95 = Less Or Equal To 0?(x=w295) -> (x <= 0?=w294:bool)
            n96 = Add(x=w301, y=w295) -> (x+y=w300:dbl)
            n97 = case shown="False" w294 {
              tunnel: w305 -> [w320 w323]
              tunnel: [w319 w324] -> w304
              tunnel: w303 -> [w318 w321]
              tunnel: w300 -> [w317 _]
              tunnel: w299 -> [w316 _]
              tunnel: w298 -> [w314 _]
              tunnel: [w312 w323] -> w297
              tunnel: w296 -> [w309 _]
              tunnel: w293 -> [w307 _]
              tunnel: w292 -> [w306 _]
              frame False {
                w311 = "%s %s"  # Format
                # "If sufficient amount"
                n98 = Number To Fractional String(number=w317) -> (F-format string=w313:string)  [unwired: 3 in]
                n99 = Format Into String(format string=w311, initial string=w307, error in=w320, w309, w306) -> (resulting string=w310:string, error out=w312:errorcluster)
                n100 = Replace Array Subset(array=w316, new element=w313, index=w314) -> (w315:string[])
                n101 = Bundle By Name(cluster=w318, "Selected_Account_Details"=w315, "ATM_Message"=w310, "Selected_Banking"="") -> (w319:T9)
              }
              frame True {
                # "If In-sufficient amount"
                n102 = Unbundle By Name(w321) -> ("ATM_Message 2.ATMM_Deposit_Insufficient"=w322:string)
                n103 = Bundle By Name(cluster=w321, "ATM_Message"=w322) -> (w324:T9)
              }
            }
          }
        }
        n104 = call "Queue_Driver.vi"("State_Data_In"=w219, "Error_In"=w222, "Queue_Operation_Select"=w220) -> ("Error_Out"=w218:errorcluster)  [unwired: 11 in, 1 out]
      }
      frame "----------Exception_Handling-----------" {
      }
      frame "Error_State" {
        w330 = T8 {"State"="Exit", "Data"=""}  # State_Data_In
        w331 = Queue_Operation_Select."Enqueue"  # Queue_Operation_Select
        w339 = "%d%s%s"  # Format_String
        w340 = "Application Error"  # Initial_String
        w341 = "Stop"  # T_Button
        w342 = "Continue"  # F_Button
        # "Handles the Error"
        n105 = call <vilib>:"Clear Errors.vi"("error in (no error)"=w333) -> ("error out"=w337:errorcluster)  [unwired: 5 in, 1 out]
        n106 = Unbundle By Name(w333) -> ("code"=w336:i32, "source"=w335:string)
        n107 = Format Into String(format string=w339, initial string=w340, error in=w337, w336, "\n", w335) -> (resulting string=w343:string, error out=w334:errorcluster)
        n108 = Two Button Dialog(message=w343, 1:w342, 2:w341) -> (T button?=w327:bool)
        n109 = Select(t=w330, s=w327, f=T8 {"State"="FP_Update", "Data"=""}) -> (s? t:f=w329:T8)
        n110 = call "Queue_Driver.vi"("State_Data_In"=w329, "Error_In"=w334, "Queue_Operation_Select"=w331) -> ("Error_Out"=w332:errorcluster)  [unwired: 11 in, 1 out]
      }
      frame "Exit" {
        w348 = "No"  # Continue_Exe
        w347 = "Yes"  # Stop_Exe
        w351 = Notifier_Operation_Select."Send_Notification"  # Notifier_Operation_Select
        # "Close the applicatiom"
        n111 = disable-structure shown="Default" {
          disable-tunnel: w350 -> [w355 w357]
          disable-tunnel: [w355 w357] -> w349
          disable-tunnel: [w354 w356] -> w346
          frame condition #0 (active) {
            w354 = "Do you want to stop the execution"  # Message
            # "Developer mode"
          }
          frame condition #1 {
            w356 = "Do you want to Exit"  # Message
            # "Real time engine mode or application mode"
          }
        }
        n112 = Two Button Dialog(message=w346, 1:w348, 2:w347) -> (T button?=w345:bool)
        n113 = call "Notifier_Driver.vi"("Notification"=w345, "Error_In"=w349, "Notifier_Operation_Select"=w351) -> ("Error_Out"=w352:errorcluster)  [unwired: 11 in, 1 out]
      }
    }
  }
  n114 = while {
    tunnel: T8 {"State"="", "Data"=""} ("State_Data_In") -> [w360]
    shift-right: [w361] -> w3
    shift-left: w13 -> [w362]
    stop <- w358 stop-if-true
    # "Producer"
    n115 = event shown="[1] \"Card_Simulator\": Value Change" {
      selector: _ -> [_ _ _ _ _ _]
      dyn-events: _ -> [_ _ _ _ _ _]
      timeout: 2 -> [_ _ _ _ _ _]
      tunnel: w362 -> [w370 w384 w388 w411 w423 w428]
      tunnel: [w365 w378 w387 w409 w414 w426] -> w361
      tunnel: w360 -> [_ _ w386 w410 w418 _]
      tunnel: [w363 _ _ _ _ _] -> w358
      event Timeout {
        w364 = Notifier_Operation_Select."Get_Notification_Status"  # Notifier_Operation_Select
        w367 = Timer_Operation_Select."Time_Out?"  # Timer_Select
        n116 = event-data() -> ()  [unwired: 1 in, 3 out]
        n117 = call "Timer.vi"("Error_In"=w370, "Timer_Select"=w367) -> ("Time_Out?"=w368:bool, "Error_Out"=w369:errorcluster)  [unwired: 12 in]
        n118 = case shown="False" w368 {
          tunnel: w369 -> [w371 w377]
          tunnel: [w371 w373] -> w366
          frame False {
          }
          frame True {
            w372 = Timer_Operation_Select."Stop_Timer"  # Timer_Select
            w375 = Queue_Operation_Select."Enqueue_N"  # Queue_Operation_Select
            n119 = call "Queue_Driver.vi"("State_Data_In_N"=T8[] [{"State"="Pre_Initialize", "Data"=""}, {"State"="Initialize", "Data"=""}, {"State"="Disable_Enable_Control", "Data"=""}, {"State"="FP_Update", "Data"=""}], "Error_In"=w377, "Queue_Operation_Select"=w375) -> ("Error_Out"=w376:errorcluster)  [unwired: 11 in, 1 out]
            n120 = call "Timer.vi"("Error_In"=w376, "Timer_Select"=w372) -> ("Error_Out"=w373:errorcluster)  [unwired: 12 in, 1 out]
          }
        }
        n121 = call "Notifier_Driver.vi"("Error_In"=w366, "Notifier_Operation_Select"=w364) -> ("Latest_Notification"=w363:bool, "Error_Out"=w365:errorcluster)  [unwired: 12 in]
      }
      event "Card_Simulator": Value Change {
        w380 = 10.0  # Time_Required
        w381 = Timer_Operation_Select."Start_Timer"  # Timer_Select
        w382 = Queue_Operation_Select."Enqueue_N"  # Queue_Operation_Select
        n122 = event-data() -> ()  [unwired: 1 in, 1 out]
        n123 = call "Queue_Driver.vi"("State_Data_In_N"=T8[] [{"State"="Card_Inserted", "Data"=""}, {"State"="Disable_Enable_Control", "Data"=""}, {"State"="FP_Update", "Data"=""}], "Error_In"=w384, "Queue_Operation_Select"=w382) -> ("Error_Out"=w383:errorcluster)  [unwired: 11 in, 1 out]
        n124 = call "Timer.vi"("Time_Required"=w380, "Error_In"=w383, "Timer_Select"=w381) -> ("Error_Out"=w378:errorcluster)  [unwired: 11 in, 1 out]
      }
      event "User_Input": Key Down {
        n125 = event-data() -> ("ScanCode"=w385:i16)  [unwired: 1 in]
        n126 = case shown="28" w385 {
          tunnel: w388 -> [w389 w392]
          tunnel: w386 -> [_ w396]
          tunnel: [w389 w395] -> w387
          frame 0, Default {
          }
          frame 28 {
            w393 = 10.0  # Time_Required
            w394 = Timer_Operation_Select."Start_Timer"  # Timer_Select
            w399 = "Enter"  # State
            w400 = Queue_Operation_Select."Enqueue"  # Queue_Operation_Select
            n127 = property on="User_Input" class="Str"(error in=w392) -> (error out=w391:errorcluster, "Value"=w390:string)  [unwired: 1 in, 1 out]
            n128 = Bundle By Name(cluster=w396, "State"=w399, "Data"=w390) -> (w397:T8)
            n129 = call "Queue_Driver.vi"("State_Data_In"=w397, "Error_In"=w391, "Queue_Operation_Select"=w400) -> ("Error_Out"=w398:errorcluster)  [unwired: 11 in, 1 out]
            n130 = call "Timer.vi"("Time_Required"=w393, "Error_In"=w398, "Timer_Select"=w394) -> ("Error_Out"=w395:errorcluster)  [unwired: 11 in, 1 out]
          }
        }
      }
      event "Enter": Value Change {
        w403 = 10.0  # Time_Required
        w404 = Timer_Operation_Select."Start_Timer"  # Timer_Select
        w407 = "Enter"  # State
        w408 = Queue_Operation_Select."Enqueue"  # Queue_Operation_Select
        n131 = event-data() -> ()  [unwired: 1 in, 1 out]
        n132 = property on="User_Input" class="Str"(error in=w411) -> (error out=w402:errorcluster, "Value"=w401:string)  [unwired: 1 in, 1 out]
        n133 = Bundle By Name(cluster=w410, "State"=w407, "Data"=w401) -> (w405:T8)
        n134 = call "Queue_Driver.vi"("State_Data_In"=w405, "Error_In"=w402, "Queue_Operation_Select"=w408) -> ("Error_Out"=w406:errorcluster)  [unwired: 11 in, 1 out]
        n135 = call "Timer.vi"("Time_Required"=w403, "Error_In"=w406, "Timer_Select"=w404) -> ("Error_Out"=w409:errorcluster)  [unwired: 11 in, 1 out]
      }
      event "Left_Buttons.None", "Left_Buttons.Balance_Inquiry", "Left_Buttons.Return_Card_&_Terminate", "Right_Buttons.Deposit", "Right_Buttons.Withdraw", "Right_Buttons.Fast_Cash_$50": Value Change {
        w412 = 10.0  # Time_Required
        w419 = Queue_Operation_Select."Enqueue"  # Queue_Operation_Select
        n136 = event-data() -> ("CtlRef"=w421:refnum<vi>)  [unwired: 1 in]
        n137 = property class="Bool"(reference=w421, error in=w423) -> (error out=w422:errorcluster, "Label.Text"=w416:string)  [unwired: 1 out]
        n138 = Bundle By Name(cluster=w418, "State"="Banking_Select", "Data"=w416) -> (w417:T8)
        n139 = call "Queue_Driver.vi"("State_Data_In"=w417, "Error_In"=w422, "Queue_Operation_Select"=w419) -> ("Error_Out"=w420:errorcluster)  [unwired: 11 in, 1 out]
        n140 = call "Timer.vi"("Time_Required"=w412, "Error_In"=w420, "Timer_Select"=Timer_Operation_Select."Start_Timer") -> ("Error_Out"=w414:errorcluster)  [unwired: 11 in, 1 out]
      }
      event Panel Close? {
        w424 = T8 {"State"="Exit", "Data"=""}  # State_Data_In
        w425 = Queue_Operation_Select."Enqueue"  # Queue_Operation_Select
        n141 = event-data() -> ()  [unwired: 1 in, 1 out]
        n142 = call "Queue_Driver.vi"("State_Data_In"=w424, "Error_In"=w428, "Queue_Operation_Select"=w425) -> ("Error_Out"=w426:errorcluster)  [unwired: 11 in, 1 out]
        n143 = event-data("Discard?"=TRUE) -> ()  [unwired: 1 in, 1 out]
      }
    }
  }
  n144 = Merge Errors(w3, w14) -> (w2:errorcluster)
  n145 = call "Timer.vi"("Error_In"=w2, "Timer_Select"=w8) -> ("Error_Out"=w9:errorcluster)  [unwired: 12 in, 1 out]
  n146 = call "Queue_Driver.vi"("Error_In"=w9, "Queue_Operation_Select"=w7) -> ("Error_Out"=w10:errorcluster)  [unwired: 12 in, 1 out]
  n147 = call "Queue_Driver.vi"("Error_In"=w10, "Queue_Operation_Select"=w5) -> ("Error_Out"=w6:errorcluster)  [unwired: 12 in, 1 out]
  n148 = call "Notifier_Driver.vi"("Error_In"=w6, "Notifier_Operation_Select"=w4) -> ("Error_Out"=→"Error_Out":errorcluster)  [unwired: 12 in, 1 out]
